vi "getDictionaryEntry.vi"(8 "error in":errorcluster, 9 "byte order":T1(ring), 10 "DE_offset":u32, 11 "tif_file":refnum<file>) -> (0 "error out":errorcluster, 3 "output cluster":T2)   [LabVIEW 2013]
panel:
  in  "Tab Control":enum32{"Page 1", "Page 2"}(tab)
  out "type1":u8[](array[numeric])
  in  "type2":string
  out "type3":u16[](array[numeric])
  out "type4":u32[](array[numeric])
  in  "type5":u32[](array[numeric])
  out "DE_data_offset":u32
  out "DE_data_num":u32
  out "tag_ID":u16 format="%x"
  out "type_ID":u16 format="%x"
  in  "type4_U32":u32
  in  "type3_U16":u16
  in  "type1_U8":u8
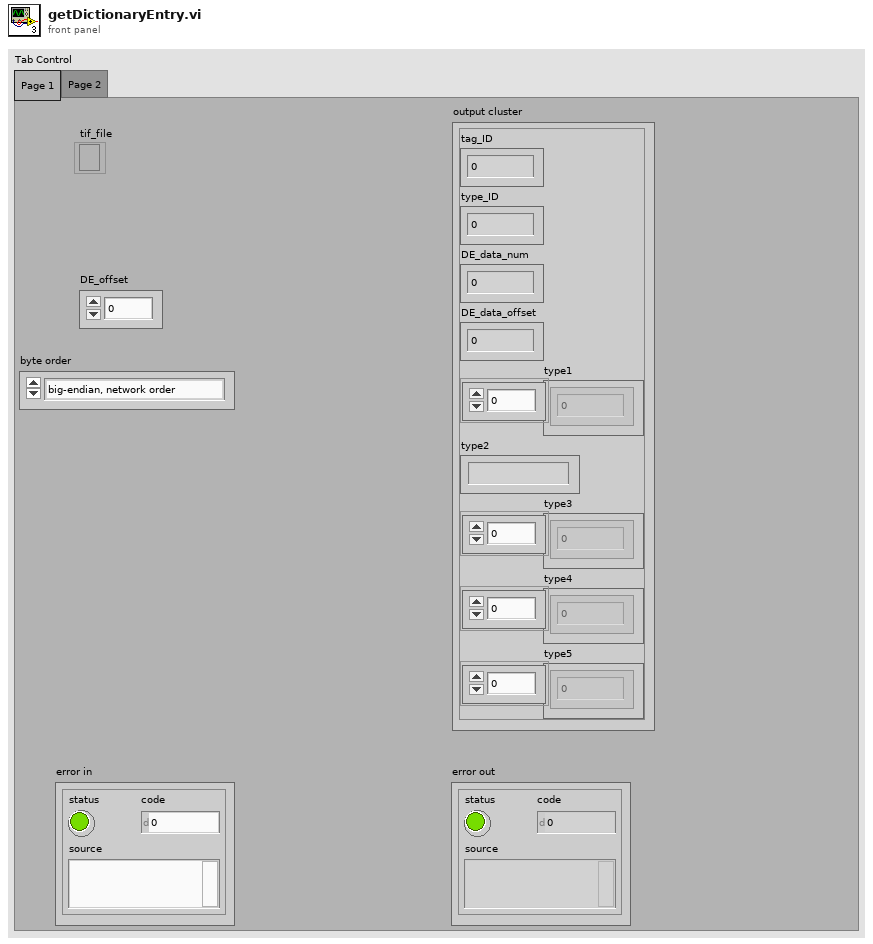
[diagram p1: front panel]
types:
  T1 = enum16{"big-endian, network order", "native, host order", "little-endian"}
  T2 = cluster{"tag_ID":u16, "type_ID":u16, "DE_data_num":u32, "DE_data_offset":u32, "type1":u8[], "type2":string, "type3":u16[], "type4":u32[], "type5":u32[]}
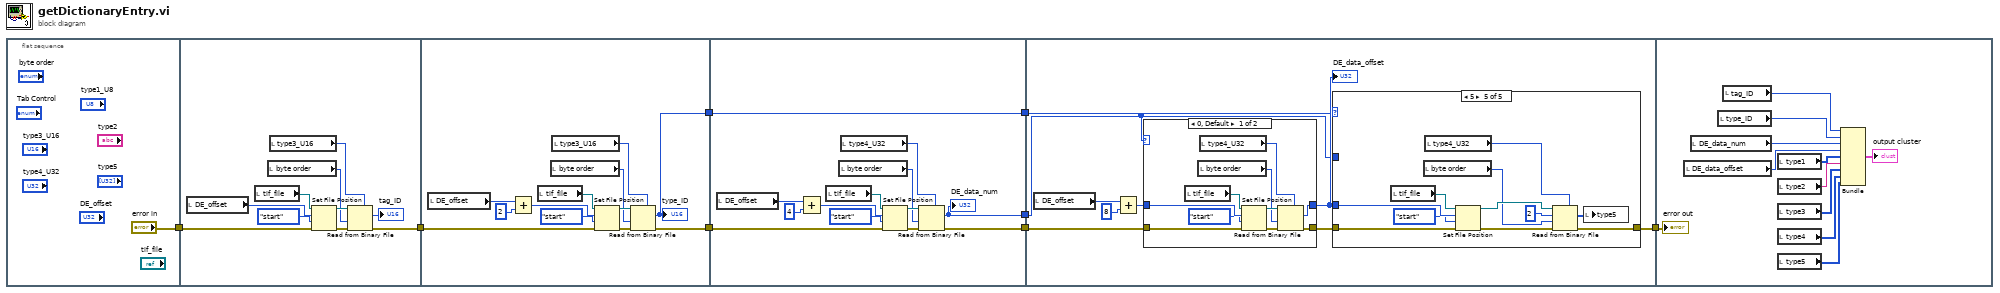
[diagram p0: block diagram]
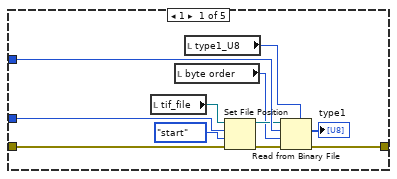
[diagram p3: hidden frame]
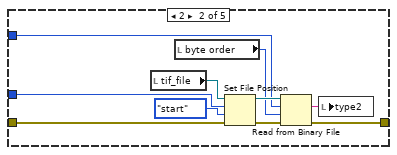
[diagram p4: hidden frame]
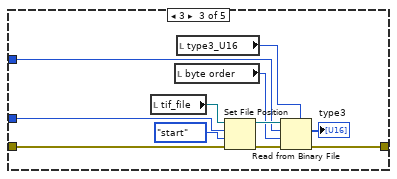
[diagram p5: hidden frame]
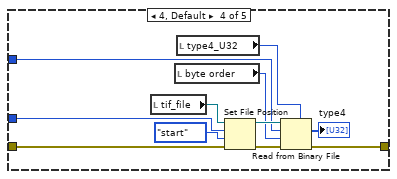
[diagram p6: hidden frame]
diagram:
  n1 = flat-sequence {
    tunnel: ["error in"] -> w5
    tunnel: w5 -> [w12]
    tunnel: [w11] -> w4
    tunnel: [w23] -> w8
    tunnel: w4 -> [w22]
    tunnel: [w21] -> w3
    tunnel: [w44] -> w7
    tunnel: w8 -> [w44]
    tunnel: [w35] -> w6
    tunnel: w3 -> [w34]
    tunnel: [w33] -> w2
    tunnel: w7 -> [w49]
    tunnel: w6 -> [w50]
    tunnel: w2 -> [w48]
    tunnel: [w46] -> w1
    tunnel: w1 -> [w130]
    frame #0 {
    }
    frame #1 {
      n2 = local read "DE_offset"() -> (w10:u32)
      n3 = local read "tif_file"() -> (w18:refnum<file>)
      n4 = local read "byte order"() -> (w14:T1)
      n5 = local read "type3_U16"() -> (w13:u16)
      n6 = Set File Position(offset (in bytes) (0)=w10, refnum=w18, from (0:start)=enum16{"start", "end", "current"}."start", error in=w12) -> (refnum out=w15:refnum<file>, error out=w16:errorcluster)
      n7 = Read from Binary File(5:w13, 8:w16, 9:w14, 11:w15) -> (0:w11:errorcluster, 2:→"tag_ID":u16)  [unwired: 2 in, 2 out]
    }
    frame #2 {
      n8 = local read "DE_offset"() -> (w20:u32)
      n9 = Add(x=w20, y=2) -> (x+y=w25:u32)
      n10 = local read "tif_file"() -> (w31:refnum<file>)
      n11 = local read "byte order"() -> (w27:T1)
      n12 = local read "type3_U16"() -> (w26:u16)
      n13 = Set File Position(offset (in bytes) (0)=w25, refnum=w31, from (0:start)=enum16{"start", "end", "current"}."start", error in=w22) -> (refnum out=w28:refnum<file>, error out=w29:errorcluster)
      n14 = Read from Binary File(5:w26, 8:w29, 9:w27, 11:w28) -> (0:w21:errorcluster, 2:w23:u16)  [unwired: 2 in, 2 out]
      "type_ID" <- w23
    }
    frame #3 {
      n15 = local read "DE_offset"() -> (w32:u32)
      n16 = Add(x=w32, y=4) -> (x+y=w36:u32)
      n17 = local read "tif_file"() -> (w43:refnum<file>)
      n18 = local read "byte order"() -> (w39:T1)
      n19 = local read "type4_U32"() -> (w38:u32)
      n20 = Set File Position(offset (in bytes) (0)=w36, refnum=w43, from (0:start)=enum16{"start", "end", "current"}."start", error in=w34) -> (refnum out=w40:refnum<file>, error out=w41:errorcluster)
      n21 = Read from Binary File(5:w38, 8:w41, 9:w39, 11:w40) -> (0:w33:errorcluster, 2:w35:u32)  [unwired: 2 in, 2 out]
      "DE_data_num" <- w35
    }
    frame #4 {
      n22 = local read "DE_offset"() -> (w45:u32)
      n23 = Add(x=w45, y=8) -> (x+y=w52:u32)
      n24 = case shown="0, Default" w50 {
        tunnel: w52 -> [w63 w65]
        tunnel: [w62 w65] -> w51
        tunnel: w48 -> [w61 w64]
        tunnel: [w60 w64] -> w47
        frame 0, Default {
          n25 = local read "tif_file"() -> (w59:refnum<file>)
          n26 = local read "byte order"() -> (w55:T1)
          n27 = local read "type4_U32"() -> (w54:u32)
          n28 = Set File Position(offset (in bytes) (0)=w63, refnum=w59, from (0:start)=enum16{"start", "end", "current"}."start", error in=w61) -> (refnum out=w56:refnum<file>, error out=w57:errorcluster)
          n29 = Read from Binary File(5:w54, 8:w57, 9:w55, 11:w56) -> (0:w60:errorcluster, 2:w62:u32)  [unwired: 2 in, 2 out]
        }
        frame 1 {
        }
      }
      "DE_data_offset" <- w51
      n30 = case shown="5" w49 {
        tunnel: w51 -> [w76 w86 w97 w108 w119]
        tunnel: w50 -> [w75 w80 w90 w101 _]
        tunnel: w47 -> [w68 w79 w89 w100 w118]
        tunnel: [w67 w78 w88 w99 w117] -> w46
        frame 1 {
          n31 = local read "tif_file"() -> (w74:refnum<file>)
          n32 = local read "byte order"() -> (w70:T1)
          n33 = local read "type1_U8"() -> (w69:u8)
          n34 = Set File Position(offset (in bytes) (0)=w76, refnum=w74, from (0:start)=enum16{"start", "end", "current"}."start", error in=w68) -> (refnum out=w71:refnum<file>, error out=w72:errorcluster)
          n35 = Read from Binary File(5:w69, 8:w72, 9:w70, 10:w75, 11:w71) -> (0:w67:errorcluster, 2:→"type1":u8[])  [unwired: 1 in, 2 out]
        }
        frame 2 {
          n36 = local read "tif_file"() -> (w85:refnum<file>)
          n37 = local read "byte order"() -> (w81:T1)
          n38 = Set File Position(offset (in bytes) (0)=w86, refnum=w85, from (0:start)=enum16{"start", "end", "current"}."start", error in=w79) -> (refnum out=w82:refnum<file>, error out=w83:errorcluster)
          n39 = Read from Binary File(8:w83, 9:w81, 10:w80, 11:w82) -> (0:w78:errorcluster, 2:w77:string)  [unwired: 2 in, 2 out]
          n40 = local write "type2"(w77) -> ()
        }
        frame 3 {
          n41 = local read "tif_file"() -> (w96:refnum<file>)
          n42 = local read "byte order"() -> (w92:T1)
          n43 = local read "type3_U16"() -> (w91:u16)
          n44 = Set File Position(offset (in bytes) (0)=w97, refnum=w96, from (0:start)=enum16{"start", "end", "current"}."start", error in=w89) -> (refnum out=w93:refnum<file>, error out=w94:errorcluster)
          n45 = Read from Binary File(5:w91, 8:w94, 9:w92, 10:w90, 11:w93) -> (0:w88:errorcluster, 2:→"type3":u16[])  [unwired: 1 in, 2 out]
        }
        frame 4, Default {
          n46 = local read "tif_file"() -> (w107:refnum<file>)
          n47 = local read "byte order"() -> (w103:T1)
          n48 = local read "type4_U32"() -> (w102:u32)
          n49 = Set File Position(offset (in bytes) (0)=w108, refnum=w107, from (0:start)=enum16{"start", "end", "current"}."start", error in=w100) -> (refnum out=w104:refnum<file>, error out=w105:errorcluster)
          n50 = Read from Binary File(5:w102, 8:w105, 9:w103, 10:w101, 11:w104) -> (0:w99:errorcluster, 2:→"type4":u32[])  [unwired: 1 in, 2 out]
        }
        frame 5 {
          n51 = local read "tif_file"() -> (w116:refnum<file>)
          n52 = local read "byte order"() -> (w112:T1)
          n53 = local read "type4_U32"() -> (w111:u32)
          n54 = Set File Position(offset (in bytes) (0)=w119, refnum=w116, from (0:start)=enum16{"start", "end", "current"}."start", error in=w118) -> (refnum out=w113:refnum<file>, error out=w114:errorcluster)
          n55 = Read from Binary File(5:w111, 8:w114, 9:w112, 10:2 ("count (1)"), 11:w113) -> (0:w117:errorcluster, 2:w109:u32[])  [unwired: 1 in, 2 out]
          n56 = local write "type5"(w109) -> ()
        }
      }
    }
    frame #5 {
      n57 = local read "DE_data_offset"() -> (w126:u32)
      n58 = local read "DE_data_num"() -> (w127:u32)
      n59 = local read "type_ID"() -> (w128:u16)
      n60 = local read "tag_ID"() -> (w129:u16)
      n61 = local read "type1"() -> (w125:u8[])
      n62 = local read "type2"() -> (w124:string)
      n63 = local read "type3"() -> (w123:u16[])
      n64 = local read "type4"() -> (w122:u32[])
      n65 = local read "type5"() -> (w121:u32[])
      n66 = Bundle("tag_ID"=w129, "type_ID"=w128, "DE_data_num"=w127, "DE_data_offset"=w126, "type1"=w125, "type2"=w124, "type3"=w123, "type4"=w122, "type5"=w121) -> (→"output cluster":T2)  [unwired: 1 in]
      "error out" <- w130
    }
  }
